vi "Activate.vi"(7 "Alarm Reason":string, 8 "error in (no error)":errorcluster, 9 "Alarm in":bool, 11 "Data Value Reference in":refnum<data-value>) -> (0 "error out":errorcluster)   [LabVIEW 2018, in "Alarm.lvclass"]
uses:
  Alarm.lvclass
  Alarm UI.vi
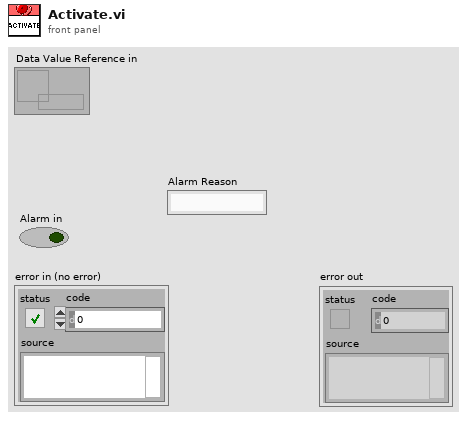
[diagram p1: front panel]
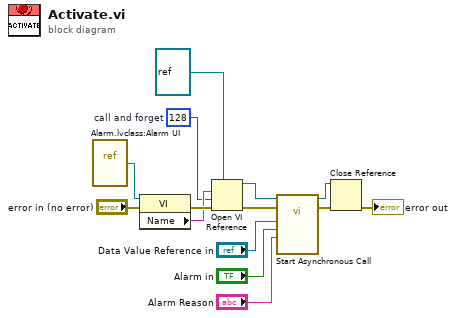
[diagram p0: block diagram]
diagram:
  w4 = 128  # call and forget
  n1 = vi-ref "Alarm.lvclass:Alarm UI.vi"() -> (w6:refnum<vi>)
  n2 = property class="VI"(reference=w6, error in="error in (no error)") -> (error out=w8:errorcluster, "Name"=w7:string)  [unwired: 1 out]
  n3 = Open VI Reference(type specifier VI Refnum (for type only)=refnum<vi> refnum, vi path=w7, options=w4, error in (no error)=w8) -> (vi reference=w3:refnum<vi>, error out=w1:errorcluster)  [unwired: 2 in]
  n4 = call-by-ref "Start Asynchronous Call"(reference=w3, error in=w1, "Alarm Reason in"="Alarm Reason", "Alarm in"="Alarm in", "Alarm DVR"="Data Value Reference in") -> (reference out=w9:refnum<vi>, error out=w10:errorcluster)  [unwired: 9 in]
  n5 = Close Reference(reference=w9, error in (no error)=w10) -> (error out=→"error out":errorcluster)
